vi "Sandbox 3 - General Testing.vi"() -> ()   [LabVIEW 2022 SP3]
uses:
  <vilib>/Utility/sysdir.llb/System Directory Type.ctl
panel:
  out "resulting string":string
  out "Public Documents":path
  out "error out":errorcluster
  out "system directory":path
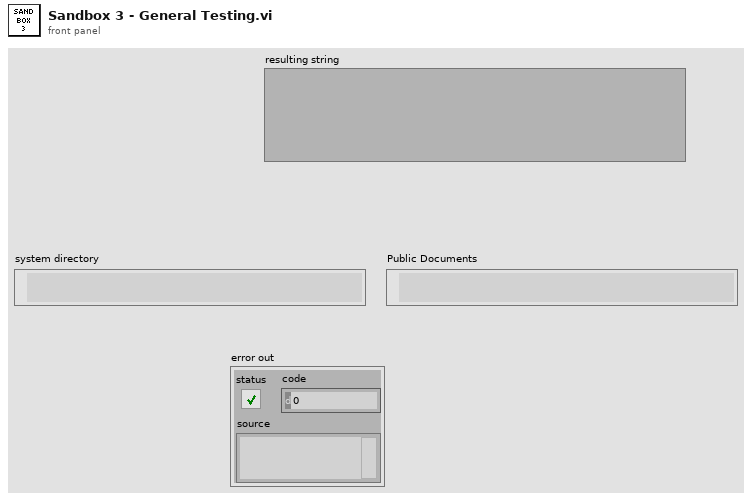
[diagram p1: front panel]
types:
  T1 = typedef "System Directory Type.ctl" = i32
  T2 = typedef "Registry RtKey.ctl" = enum32{"HKEY_CLASSES_ROOT", "HKEY_CURRENT_USER", "HKEY_LOCAL_MACHINE", "HKEY_USERS", "HKEY_PERFORMANCE_DATA", "HKEY_CURRENT_CONFIG", "HKEY_DYN_DATA"}
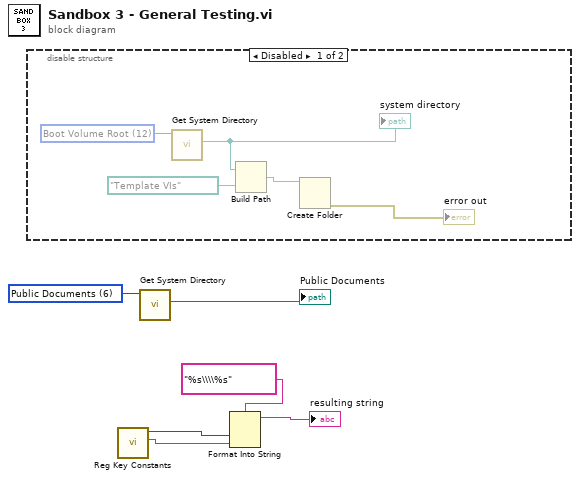
[diagram p0: block diagram]
diagram:
  w6 = T1 6 items=["User Home"=0, "User Desktop"=1, "User Documents"=2, "User Application Data"=3, "User Preferences"=4, "User Temporary"=5, "Public Documents"=6, "Public Application Data"=7, "Public Preferences"=8, "Public Cache"=13, "System Core Libraries"=9, "System Installed Libraries"=10, "Application Files"=11, "Boot Volume Root"=12] ("system directory type")
  n1 = disable-structure shown="Disabled" {
    frame Disabled {
      w11 = T1 12 items=["User Home"=0, "User Desktop"=1, "User Documents"=2, "User Application Data"=3, "User Preferences"=4, "User Temporary"=5, "Public Documents"=6, "Public Application Data"=7, "Public Preferences"=8, "Public Cache"=13, "System Core Libraries"=9, "System Installed Libraries"=10, "Application Files"=11, "Boot Volume Root"=12] ("system directory type")
      n2 = call <vilib>:"Get System Directory.vi"("system directory type"=w11) -> ("system directory"=w10:path)  [unwired: 10 in]
      "system directory" <- w10
      n3 = Build Path(base path=w10, name or relative path=path "Template VIs") -> (appended path=w8:path)
      n4 = Create Folder(path (use dialog)=w8) -> (error out=→"error out":errorcluster)  [unwired: 2 in, 2 out]
    }
    frame Enabled {
    }
  }
  n5 = call "Reg Key Constants.vi"() -> ("Subkey Path"=w3:string, "Root Key"=w4:T2)  [unwired: 4 in, 2 out]
  n6 = call <vilib>:"Get System Directory.vi"("system directory type"=w6) -> ("system directory"=→"Public Documents":path)  [unwired: 10 in]
  n7 = Format Into String(format string="%s\\\\%s", w4, w3) -> (resulting string=→"resulting string":string)  [unwired: 2 in, 1 out]
